vi "Solve2.vi"(8 "Error In":errorcluster, 11 "object in":refnum<class "2025_1.lvclass">) -> (0 "Error Out":errorcluster, 2 "Result":u64, 3 "object out":refnum<class "2025_1.lvclass">)   [LabVIEW 2023, in "2025_1.lvclass"]
uses:
  2025_1.lvclass
  2025_1.lvclass/2025_1.ctl
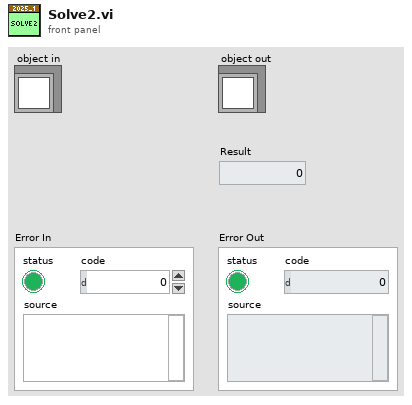
[diagram p1: front panel]
types:
  T1 = typedef "2025_1.lvclass/Turns.ctl" = cluster{"Direction":T2, "Steps":i64}
  T2 = typedef "2025_1.lvclass/Direction.ctl" = enum16{"Left", "Right"}
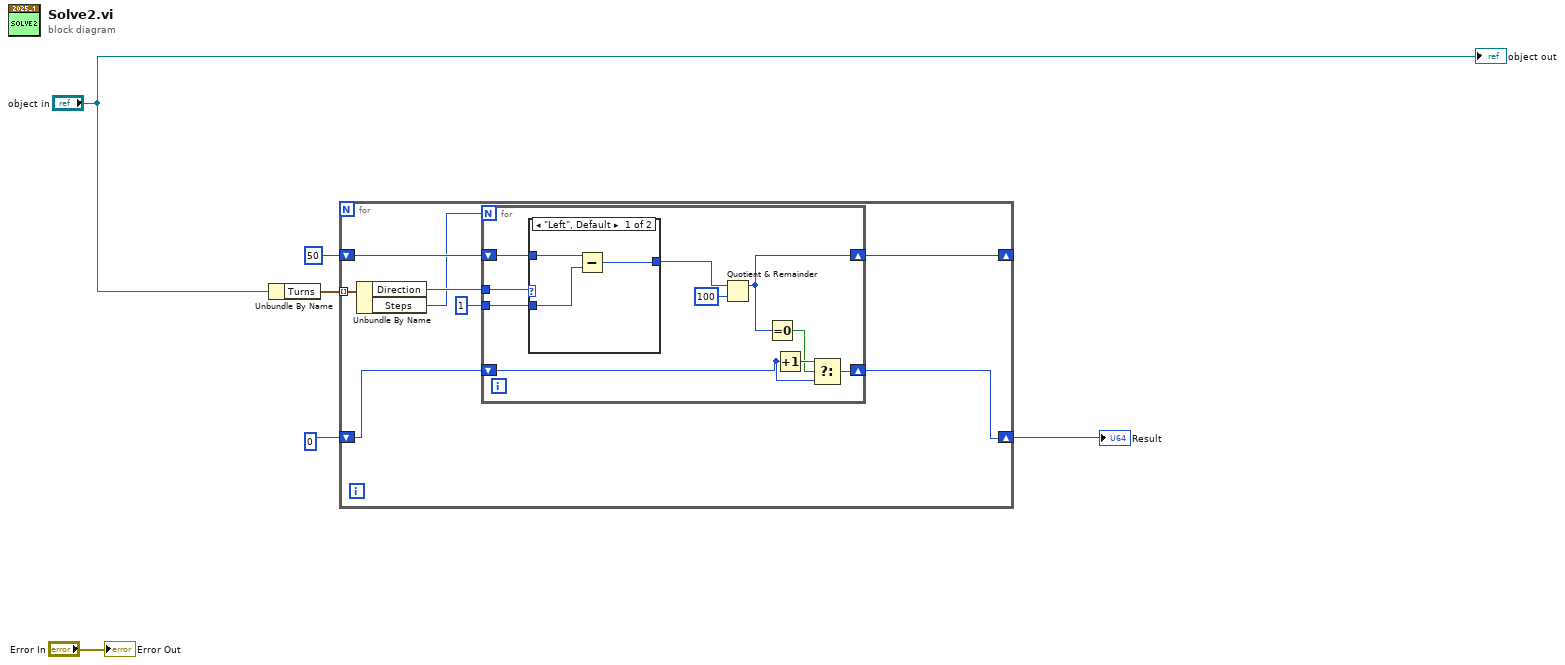
[diagram p0: block diagram]
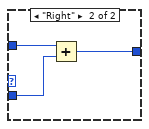
[diagram p2: hidden frame]
diagram:
  n1 = Unbundle By Name("object in") -> ("Turns"=w5:T1[])
  n2 = for {
    tunnel: w5 -> [w14] mode=indexing
    shift-right: [w11] -> _
    shift-left: i64 50 -> [w12]
    shift-right: [w7] -> w1
    shift-left: i64 0 -> [w8]
    n3 = Unbundle By Name(w14) -> ("Direction"=w13:T2, "Steps"=w10:i64)
    n4 = for {
      N: w10 -> [_]
      tunnel: w13 -> [w24]
      tunnel: i64 1 -> [w22]
      shift-right: [w19] -> w11
      shift-left: w12 -> [w23]
      shift-right: [w15] -> w7
      shift-left: w8 -> [w16]
      n5 = case shown="\"Left\", Default" w24 {
        tunnel: w23 -> [w27 w30]
        tunnel: [w25 w29] -> w20
        tunnel: w22 -> [w26 w28]
        frame "Left", Default {
          n6 = Subtract(x=w27, y=w26) -> (x-y=w25:i64)
        }
        frame "Right" {
          n7 = Add(x=w30, y=w28) -> (x+y=w29:i64)
        }
      }
      n8 = Quotient & Remainder(x=w20, y=i64 100) -> (x-y*floor(x/y)=w19:i64)  [unwired: 1 out]
      n9 = Equal To 0?(x=w19) -> (x = 0?=w17:bool)
      n10 = Increment(x=w16) -> (x+1=w18:i64)
      n11 = Select(t=w18, s=w17, f=w16) -> (s? t:f=w15:i64)
    }
  }
  "Result" <- w1
  "Error Out" <- "Error In"
  "object out" <- "object in"
